vi "Display Images.vi"(0 "fpga interface in":refnum<k20>, 1 "'stop' notifier":refnum<notifier>, 2 "rate references":T1, 5 "display channel number":i32, 7 "raw display notifier":refnum<notifier>, 9 "display reference":refnum<vi>, 11 "error in (no error)":errorcluster) -> (4 "fpga interface out":refnum<k20>, 15 "error out":errorcluster)   [LabVIEW 2023, in "GettingStarted_Common_148X_Host.lvlib"]
uses:
  GettingStarted_Common_148X_Host.lvlib
  <vilib>/rvi/interface/nirviReadWriteControl/nirviReadWriteControl.xnode
  Types/148x_Common_FPGA_Reference.ctl
  NiFpgaLv.dll
  <vilib>/Utility/error.llb/Error Cluster From Error Code.vi
  <vilib>/rvi/interface/Simulation/niFpgaSimulationCallBeginRW.vi
  <vilib>/rvi/errors/niLvFpgaAdjustHostInterfaceError.vi
  <vilib>/vision/Image Controls.llb/IMAQ Image.ctl
  Types/Serial Channel Display Parameters.ctl
  Types/RAW Interpretation for Display.ctl
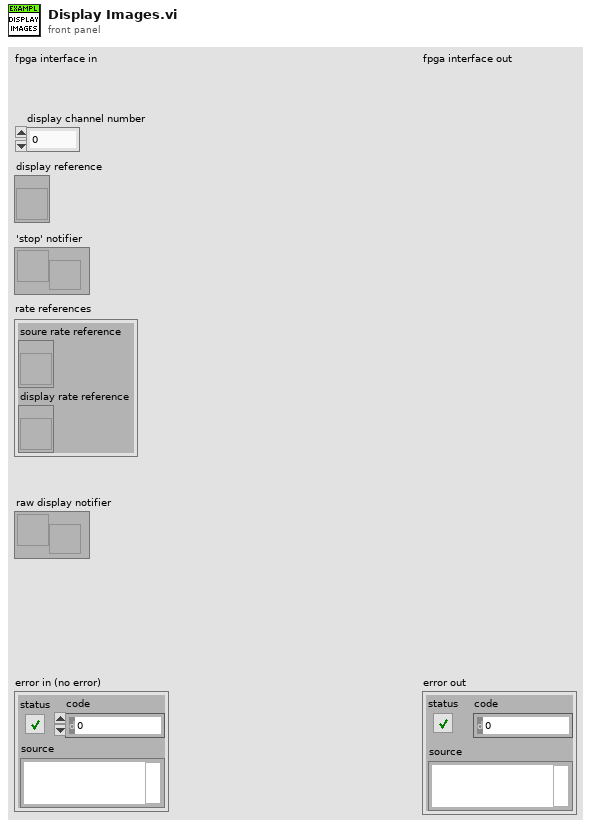
[diagram p1: front panel]
types:
  T1 = cluster{"soure rate reference":refnum<vi>, "display rate reference":refnum<vi>}
  T2 = typedef "GettingStarted_Common_148X_Host.lvlib/148x_Common_FPGA_Reference.ctl" = refnum<k20>
  T3 = typedef "GettingStarted_Common_148X_Host.lvlib/Serial Channel Display Parameters.ctl" = cluster{"images":cluster{"grayscale":T4, "color":T4}, "RAW parameters":cluster{"interpretation":T5, "bayer parameters":cluster{"pattern":i32, "algorithm":i32, "red gain":dbl, "green gain":dbl, "blue gain":dbl}}}
  T4 = typedef "IMAQ Image.ctl" = refnum<image>
  T5 = typedef "GettingStarted_Common_148X_Host.lvlib/RAW Interpretation for Display.ctl" = enum16{"Grayscale", "Bayer", "RGB", "YUV422", "YUV420", "Legacy YUV420"}
  T6 = typedef "GettingStarted_Common_148X_FPGA.lvlib/Image Metadata.ctl" = cluster{"serial channel":fxp<+,3,3>, "frame number":u16, "data type":T7, "width":u16, "height":u16, "image bytes":u32, "total bytes":u32, "little endian":bool}
  T7 = typedef "NI CSI-2 API Common v2.lvlib/LLP Data Type.ctl" = enum8{"Frame Start", "Frame End", "Line Start", "Line End", "End of Transmission", "Reserved 0", "Reserved 1", "Reserved 2", "Generic Short Packet 1", "Generic Short Packet 2", "Generic Short Packet 3", "Generic Short Packet 4", "Generic Short Packet 5", "Generic Short Packet 6", "Generic Short Packet 7", "Generic Short Packet 8", "Null", "Blanking Data", "Embedded 8-bit non Image Data", "Generic Long Packet 1", "Generic Long Packet 2", "Generic Long Packet 3", "Generic Long Packet 4", "Reserved 3", "YUV420 8-bit", "YUV420 10-bit", "Legacy YUV420 8-bit", "Reserved 4", "YUV420 8-bit Chroma Shifted", "YUV420 10-bit Chroma Shifted", "YUV422 8-bit", "YUV422 10-bit", "RGB444", "RGB555", "RGB565", "RGB666", "RGB888", "Reserved 5", "Reserved 6", "RAW 24", "RAW 6", "RAW 7", "RAW 8", "RAW 10", "RAW 12", "RAW 14", "RAW 16", "RAW 20", "User Defined 8-bit Data 1", "User Defined 8-bit Data 2", "User Defined 8-bit Data 3", "User Defined 8-bit Data 4", "User Defined 8-bit Data 5", "User Defined 8-bit Data 6", "User Defined 8-bit Data 7", "User Defined 8-bit Data 8", "USL Command", "Reserved 7", "Reserved 8", "Reserved 9", "Reserved 10", "Reserved 11", "Reserved 12", "LRTE EPD Spacer"}
  T8 = cluster{"image pixel data fifo overflow":bool, "image metadata fifo overflow":bool}[]
  T9 = cluster{"image pixel data fifo overflow":bool, "image metadata fifo overflow":bool}
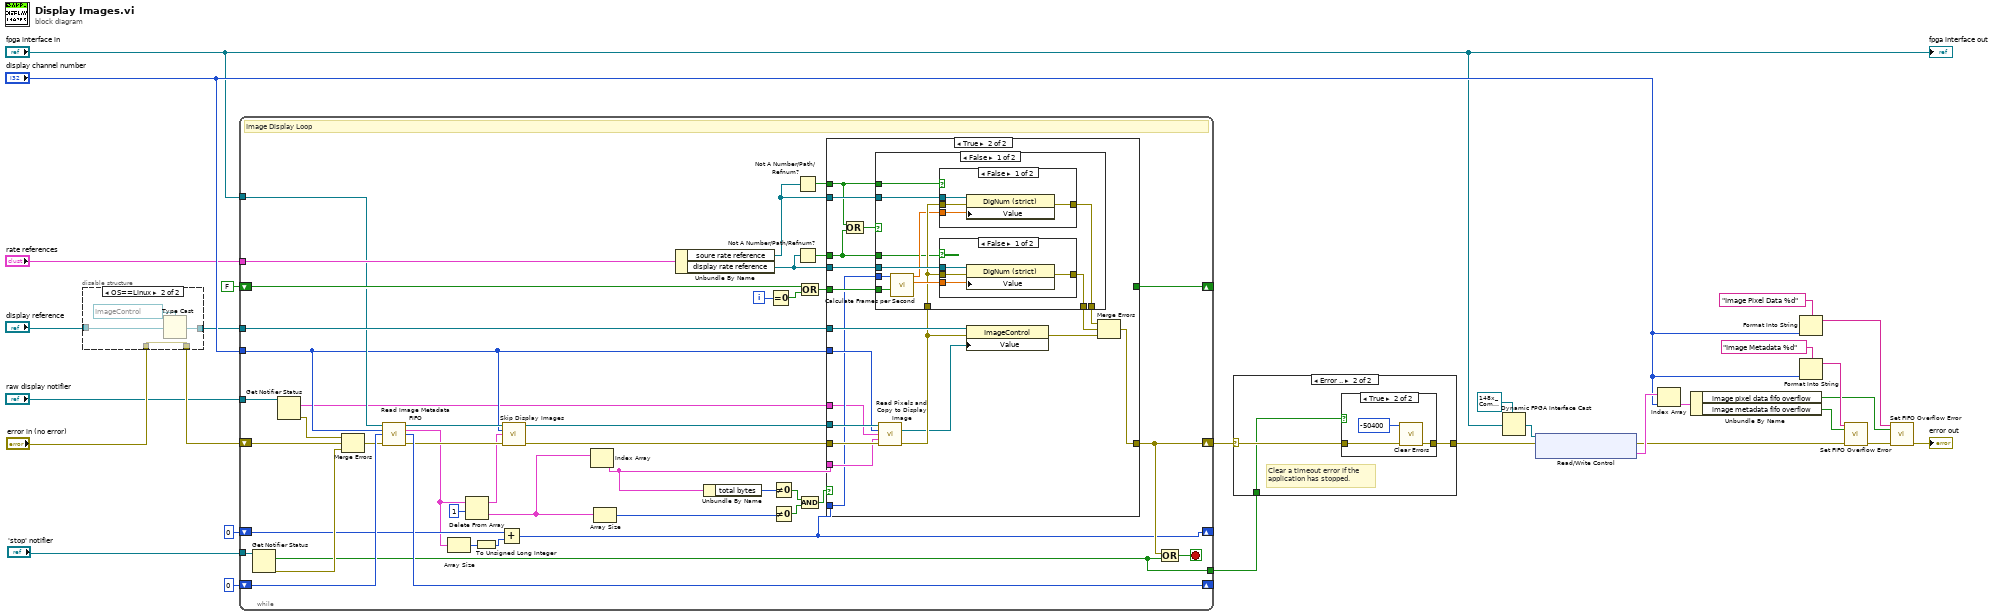
[diagram p0: block diagram]
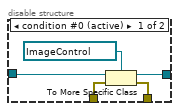
[diagram p2: hidden frame]
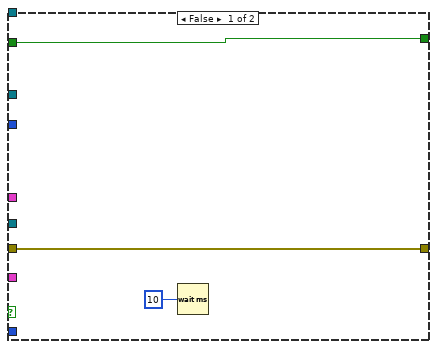
[diagram p3: hidden frame]
diagram:
  n1 = disable-structure shown="OS==Linux" {
    disable-tunnel: "display reference" -> [w32 w35]
    disable-tunnel: "error in (no error)" -> [w29 w36]
    disable-tunnel: [w31 w34] -> w5
    disable-tunnel: [w30 w36] -> w4
    frame condition #0 (active) {
      n2 = To More Specific Class(target class=refnum<vi> refnum ("reference"), reference=w32, error in=w29) -> (specific class reference=w31:refnum<vi>, error out=w30:errorcluster)
    }
    frame condition #1 {
      n3 = Type Cast(type=refnum<vi> refnum ("reference"), x=w35) -> (*(type *) &x=w34:refnum<vi>)
    }
  }
  n4 = while {
    shift-right: [w77] -> w9
    shift-left: w4 -> [w42]
    tunnel: "fpga interface in" -> [w46]
    shift-right: [w78] -> _
    shift-left: u32 0 ("Elements Remaining") -> [w65]
    tunnel: "display channel number" -> [w41]
    tunnel: w5 -> [w76]
    tunnel: "rate references" -> [w52]
    shift-right: [w69] -> _
    shift-left: FALSE -> [w66]
    shift-right: [w53] -> _
    shift-left: u32 0 ("Elements Remaining") -> [w56]
    tunnel: [w44] -> w3
    tunnel: "'stop' notifier" -> [w45]
    tunnel: "raw display notifier" -> [w40]
    i -> [w75]
    stop <- w79 stop-if-true
    # "Image Display Loop"
    n5 = Get Notifier Status(notifier=w45) -> (current notification=w44:bool, error out=w80:errorcluster)  [unwired: 1 in, 3 out]
    n6 = Get Notifier Status(notifier=w40) -> (current notification=w39:T3[], error out=w38:errorcluster)  [unwired: 1 in, 3 out]
    n7 = Merge Errors(w38, w42, w80) -> (w43:errorcluster)
    n8 = call "Read Image Metadata FIFO.vi"("fpga inteface in"=w46, "display channel number"=w41, "number of images"=w65, "error in (no error)"=w43) -> ("fpga interface out"=w61:refnum<k20>, "image metadata"=w47:T6[], "images remaining"=w78:u32, "error out"=w58:errorcluster)  [unwired: 8 in]
    n9 = Array Size(array=w47) -> (size(s)=w55:i32)
    n10 = Delete From Array(array=w47, length=1) -> (deleted portion=w62:T6[], array with subset deleted=w57:T6[])  [unwired: 1 in]
    n11 = To Unsigned Long Integer(number=w55) -> (unsigned 32bit integer=w54:u32)
    n12 = Add(x=w56, y=w54) -> (x+y=w53:u32)
    n13 = call "Skip Display Images.vi"("fpga interface in"=w61, "display channel number"=w41, "image metadata"=w57, "error in (no error)"=w58) -> ("fpga interface out"=w60:refnum<k20>, "error out"=w59:errorcluster)  [unwired: 10 in]
    n14 = Index Array(array=w62) -> (element=w74:T6)  [unwired: 1 in]
    n15 = Array Size(array=w62) -> (size(s)=w64:i32)
    n16 = Unbundle By Name(w52) -> ("soure rate reference"=w50:refnum<vi>, "display rate reference"=w51:refnum<vi>)
    n17 = Unbundle By Name(w74) -> ("total bytes"=w73:u32)
    n18 = Equal To 0?(x=w75) -> (x = 0?=w67:bool)
    n19 = Not Equal To 0?(x=w73) -> (x != 0?=w71:bool)
    n20 = Not Equal To 0?(x=w64) -> (x != 0?=w72:bool)
    n21 = Not A Number/Path/Refnum?(number/path/refnum=w50) -> (NaN/Path/Refnum?=w48:bool)
    n22 = Not A Number/Path/Refnum?(number/path/refnum=w51) -> (NaN/Path/Refnum?=w49:bool)
    n23 = Compound Arithmetic op=OR(w66, w67) -> (w68:bool)
    n24 = Compound Arithmetic op=AND(w71, w72) -> (w70:bool)
    n25 = case shown="True" w70 {
      tunnel: w59 -> [w83 w102]
      tunnel: w60 -> [_ w101]
      tunnel: w39 -> [_ w84]
      tunnel: w41 -> [_ w100]
      tunnel: [w83 w96] -> w77
      tunnel: w76 -> [_ w98]
      tunnel: w74 -> [_ w97]
      tunnel: w68 -> [w81 w93]
      tunnel: w51 -> [_ w94]
      tunnel: [w81 _] -> w69
      tunnel: w53 -> [_ w92]
      tunnel: w50 -> [_ w90]
      tunnel: w49 -> [_ w87]
      tunnel: w48 -> [_ w86]
      frame False {
        n26 = Wait (ms)(milliseconds to wait=u32 10) -> ()  [unwired: 1 out]
      }
      frame True {
        n27 = Compound Arithmetic op=OR(w86, w87) -> (w88:bool)
        n28 = call "Read Pixels and Copy to Display Image.vi"("fpga interface in"=w101, "display channel number"=w100, "serial channel display parameters"=w84, "image metadata"=w97, "error in (no error)"=w102) -> ("display image"=w85:T4, "error out"=w91:errorcluster)  [unwired: 8 in, 1 out]
        n29 = case shown="False" w88 {
          tunnel: [w113 _] -> w95
          tunnel: w94 -> [w112 _]
          tunnel: w93 -> [w111 _]
          tunnel: w92 -> [w110 _]
          tunnel: w91 -> [w108 _]
          tunnel: w90 -> [w106 _]
          tunnel: [w105 _] -> w89
          tunnel: w87 -> [w104 _]
          tunnel: w86 -> [w103 _]
          frame False {
            n30 = call <vilib>:"Calculate Frames per Second.vi"("Reset"=w111, "Buffer Number"=w110) -> ("Processed Frames/s"=w109:dbl, "Acquired Frames/s"=w107:dbl)  [unwired: 7 in, 1 out]
            n31 = case shown="False" w103 {
              tunnel: [w117 _] -> w105
              tunnel: w106 -> [w116 _]
              tunnel: w107 -> [w115 _]
              tunnel: w108 -> [w114 _]
              frame False {
                n32 = property class="DigNum (strict)"(reference=w116, error in=w114, "Value"=w115) -> (error out=w117:errorcluster)  [unwired: 1 out]
              }
              frame True {
              }
            }
            n33 = case shown="False" w104 {
              tunnel: w108 -> [w121 _]
              tunnel: [w120 _] -> w113
              tunnel: w112 -> [w119 _]
              tunnel: w109 -> [w118 _]
              frame False {
                n34 = property class="DigNum (strict)"(reference=w119, error in=w121, "Value"=w118) -> (error out=w120:errorcluster)  [unwired: 1 out]
              }
              frame True {
              }
            }
          }
          frame True {
          }
        }
        n35 = property class="ImageControl"(reference=w98, error in=w91, "Value"=w85) -> (error out=w99:errorcluster)  [unwired: 1 out]
        n36 = Merge Errors(w89, w95, w99) -> (w96:errorcluster)
      }
    }
    n37 = Compound Arithmetic op=OR(w77, w44) -> (w79:bool)
  }
  n38 = case shown="Error .." w9 {
    selector: w9 -> [w122 w125]
    tunnel: [w122 w124] -> w23
    tunnel: w3 -> [_ w123]
    frame No Error {
    }
    frame Error {
      # "Clear a timeout error if the application has stopped."
      n39 = case shown="True" w123 {
        tunnel: w125 -> [w126 w129]
        tunnel: [w126 w127] -> w124
        frame False {
        }
        frame True {
          n40 = call <vilib>:"Clear Errors.vi"("error in (no error)"=w129, "specific error code to clear (0: all)"=-50400 ("y")) -> ("error out"=w127:errorcluster)  [unwired: 4 in, 1 out]
        }
      }
    }
  }
  n41 = Dynamic FPGA Interface Cast(Session In=T2 refnum ("FPGA VI Reference Out"), Type="fpga interface in") -> (Session Out=w24:T2)
  n42 = xnode "Read/Write Control"("FPGA VI Reference In"=w24, "error in"=w23) -> ("error out"=w22:errorcluster, "display channel status"=w26:T8)  [unwired: 1 out]
  n43 = Index Array(array=w26, index="display channel number") -> (element=w27:T9)
  n44 = Unbundle By Name(w27) -> ("image pixel data fifo overflow"=w14:bool, "image metadata fifo overflow"=w13:bool)
  n45 = Format Into String(format string="Image Pixel Data %d", "display channel number") -> (resulting string=w16:string)  [unwired: 2 in, 1 out]
  n46 = Format Into String(format string="Image Metadata %d", "display channel number") -> (resulting string=w15:string)  [unwired: 2 in, 1 out]
  n47 = call "Set FIFO Overflow Error.vi"("fifo name"=w15, "overflow"=w13, "error in (no error)"=w22) -> ("error out"=w18:errorcluster)  [unwired: 12 in]
  n48 = call "Set FIFO Overflow Error.vi"("fifo name"=w16, "overflow"=w14, "error in (no error)"=w18) -> ("error out"=→"error out":errorcluster)  [unwired: 12 in]
  "fpga interface out" <- "fpga interface in"
